vi "PID_feedback_knee.vi"(4 "Reintialize":bool[](array[boolean]), 5 "currentT":dbl[](array[numeric]), 6 "dt (s)":dbl=-1.0 format="%.3f", 7 "LimitLogicIn":bool[](array[boolean]), 9 "SetTension":dbl[](array[numeric]), 10 "PID_OP_Lim":cluster{"output high":dbl, "output low":dbl}[](array[cluster])=[{"output high"=100.0, "output low"=-100.0}] {"output low" format="%.2f"; "output high" format="%.2f"}, 11 "Constants LL":T1) -> (1 "pidOP":dbl[](array[numeric]), 3 "limit logic out":bool[](array[boolean]))   [LabVIEW 2017]
uses:
  typeDef/constants_LL.ctl
  <vilib>/addons/control/pid/pid.llb/PID Advanced (DBL Array).vi
  <vilib>/addons/control/pid/pid.llb/PID Parameter Manager (DBL Array).vi
  <vilib>/addons/control/pid/pid.llb/PID Derivative Action Buffered (DBL Array).vi
  <vilib>/addons/control/pid/pid.llb/PID Get Advanced Error (DBL Array).vi
  <vilib>/addons/control/pid/pid.llb/PID Integral Action Buffered (DBL Array).vi
  <vilib>/addons/control/pid/pid.llb/PID Resize 1D Array.vi
  <vilib>/addons/control/pid/pid.llb/PID Get Advanced Error (DBL).vi
  <vilib>/addons/control/pid/NI_PID_pid.lvlib
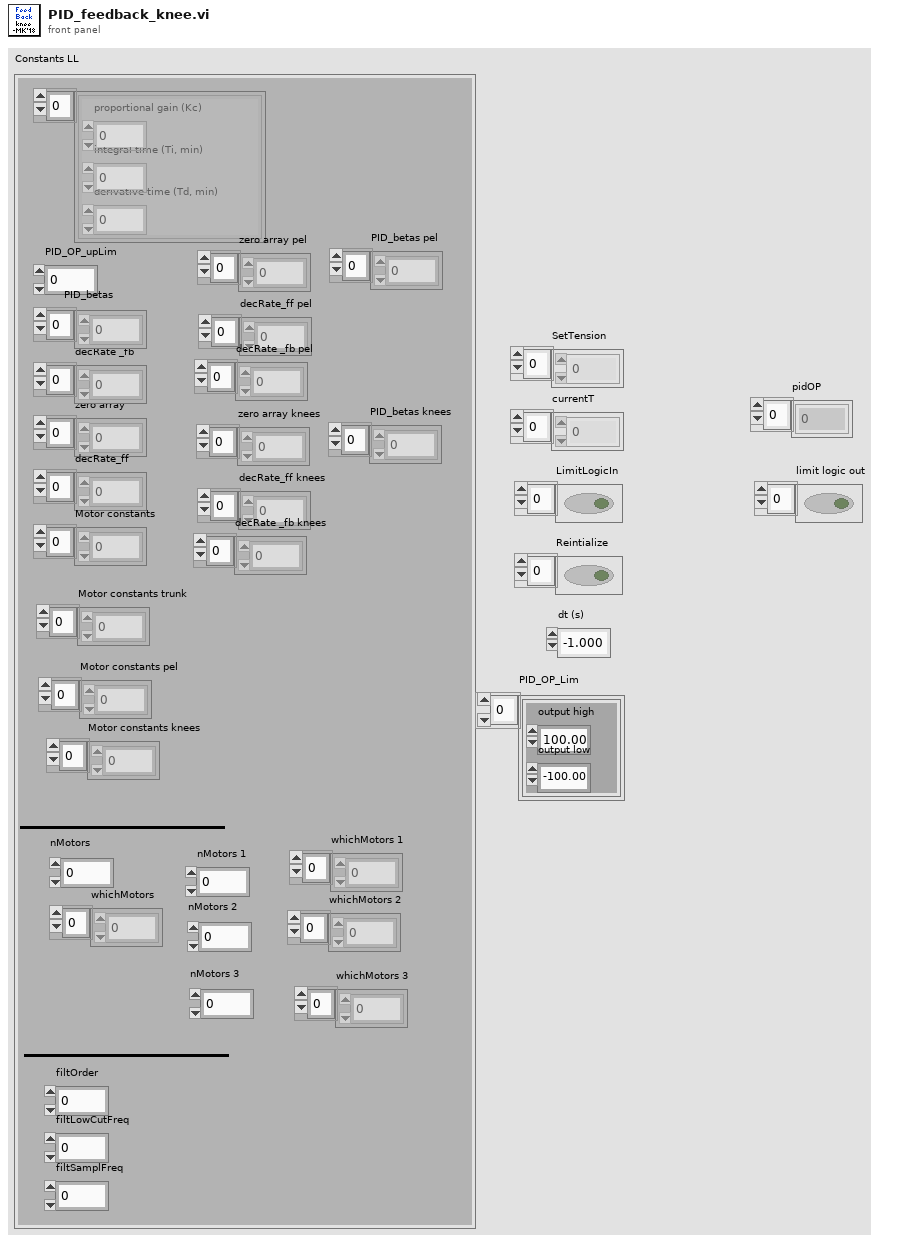
[diagram p1: front panel]
types:
  T1 = typedef "constants_LL.ctl" = cluster{"zero array":dbl[], "decRate_ff":dbl[], "Motor constants":dbl[], "PID gains":cluster{"proportional gain (Kc)":dbl, "integral time (Ti, min)":dbl, "derivative time (Td, min)":dbl}[], "decRate _fb":dbl[], "PID_OP_upLim":dbl, "nMotors":i32, "PID_betas":dbl[], "filtOrder":i32, "filtLowCutFreq":dbl, "filtSamplFreq":dbl, "whichMotors":i32[], "nMotors 1":i32, "nMotors 2":i32, "Motor constants pel":dbl[], "Motor constants trunk":dbl[], "whichMotors 1":i32[], "whichMotors 2":i32[], "zero array pel":dbl[], "decRate_ff pel":dbl[], "decRate _fb pel":dbl[], "PID_betas pel":dbl[], "whichMotors 3":i32[], "nMotors 3":i32, "Motor constants knees":dbl[], "zero array knees":dbl[], "decRate_ff knees":dbl[], "decRate _fb knees":dbl[], "PID_betas knees":dbl[]}
  T2 = cluster{"proportional gain (Kc)":dbl, "integral time (Ti, min)":dbl, "derivative time (Td, min)":dbl}[]
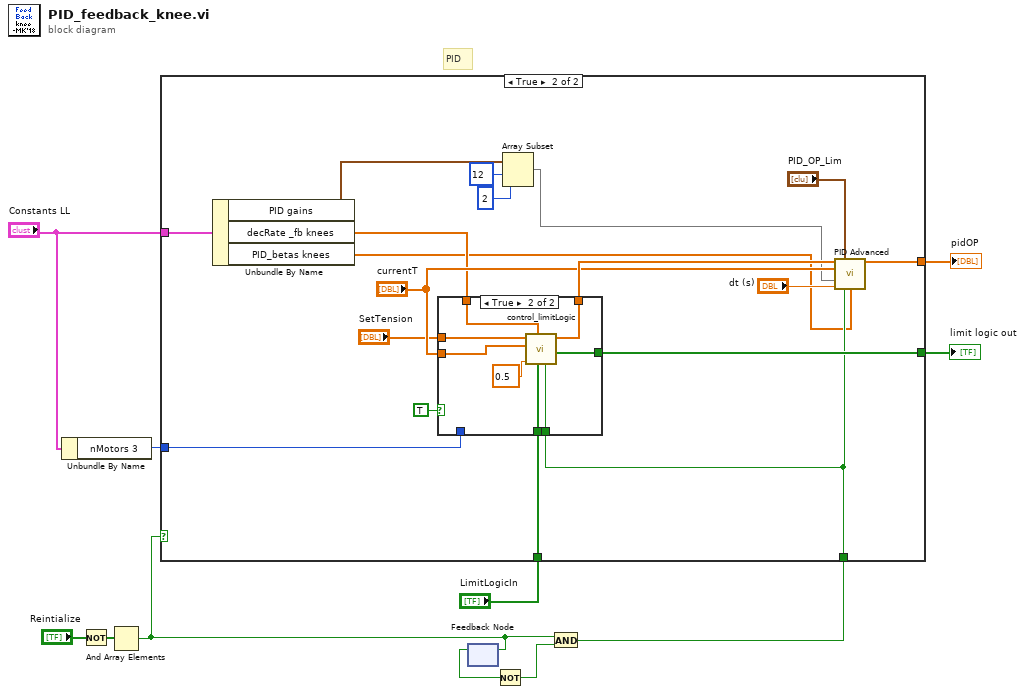
[diagram p0: block diagram]
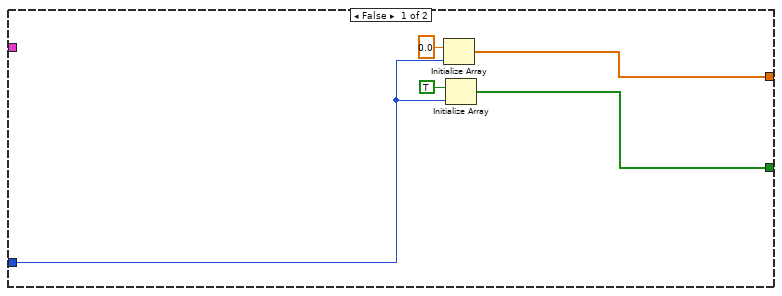
[diagram p2: hidden frame]
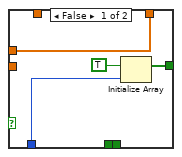
[diagram p3: hidden frame]
diagram:
  # "PID"
  n1 = Unbundle By Name("Constants LL") -> ("nMotors 3"=w1:i32)
  n2 = Not(x="Reintialize") -> (.not. x?=w7:bool[])
  n3 = And Array Elements(Boolean array=w7) -> (logical AND=w9:bool)
  n4 = feedback #1() -> (w4:bool)  [unwired: 1 in]
  n5 = feedback-in #1(w9) -> ()
  n6 = Not(x=w4) -> (.not. x?=w3:bool)
  n7 = And(x=w9, y=w3) -> (x .and. y?=w6:bool)
  n8 = case shown="True" w9 {
    tunnel: [w15 w32] -> w5
    tunnel: w6 -> [_ w31]
    tunnel: "LimitLogicIn" -> [_ w34]
    tunnel: [w13 w33] -> w11
    tunnel: w1 -> [w12 w27]
    tunnel: "Constants LL" -> [_ w28]
    frame False {
      n9 = Initialize Array(0.0 ("element"), w12) -> (w15:dbl[])
      n10 = Initialize Array(TRUE, w12) -> (w13:bool[])
    }
    frame True {
      n11 = Unbundle By Name(w28) -> ("PID gains"=w18:T2, "decRate _fb knees"=w24:dbl[], "PID_betas knees"=w23:dbl[])
      n12 = case shown="True" TRUE {
        tunnel: w31 -> [_ w46]
        tunnel: w34 -> [_ w45]
        tunnel: [w36 w44] -> w33
        tunnel: w24 -> [_ w43]
        tunnel: "SetTension" -> [w38 w42]
        tunnel: [w38 w41] -> w30
        tunnel: "currentT" -> [_ w40]
        tunnel: w27 -> [w35 _]
        frame False {
          n13 = Initialize Array(TRUE, w35) -> (w36:bool[])
        }
        frame True {
          n14 = call "control_limitLogic.vi"("reinitialize"=w46, "limit logic in"=w45, "dec rate"=w43, "diff"=0.5 ("y"), "Initial op"=w40, "Input"=w42) -> ("limit logic out"=w44:bool[], "output"=w41:dbl[])  [unwired: 4 in]
        }
      }
      n15 = Array Subset(array=w18, index=12, length=2) -> (w17:T2)
      n16 = call-poly <vilib>:"PID Advanced.vi"("setpoint"=w30, "output range"="PID_OP_Lim", "process variable"="currentT", "PID gains"=w17, "dt (s)"="dt (s)", "reinitialize? (F)"=w31, "beta"=w23) -> ("output"=w32:dbl[])  [unwired: 7 in, 1 out]
    }
  }
  "limit logic out" <- w11
  "pidOP" <- w5
